vi "Initialize Global Stop.vi"(8 "error in":errorcluster, 11 "VS Plugin Inline Async API in":refnum<class "VS Plugin Inline Async API.lvclass">) -> (0 "error out":errorcluster, 3 "VS Plugin Inline Async API out":refnum<class "VS Plugin Inline Async API.lvclass">)   [LabVIEW 2024, in "VS Plugin Inline Async API.lvlib" / "VS Plugin Inline Async API.lvclass"]
uses:
  VS Plugin Inline Async API.lvclass
  VS Plugin Inline Async API.lvclass/VS Plugin Inline Async API.ctl
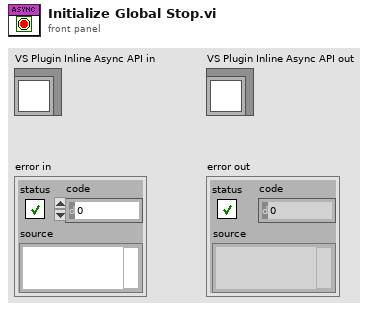
[diagram p1: front panel]
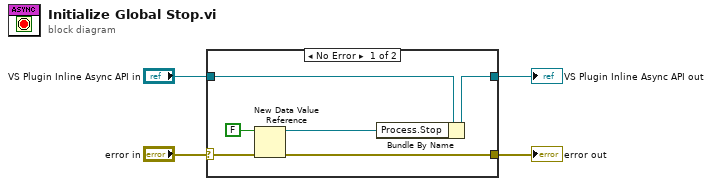
[diagram p0: block diagram]
diagram:
  n1 = case shown="No Error" "error in" {
    selector: "error in" -> [w10 w12]
    tunnel: [w9 w12] -> w3
    tunnel: "VS Plugin Inline Async API in" -> [w7 w11]
    tunnel: [w6 w11] -> w1
    frame No Error {
      n2 = New Data Value Reference(data value=FALSE, error in=w10) -> (data value reference=w5:refnum<data-value>, error out=w9:errorcluster)
      n3 = Bundle By Name(cluster=w7, "Process.Stop"=w5) -> (w6:refnum<class "VS Plugin Inline Async API.lvclass">)
    }
    frame Error {
    }
  }
  "error out" <- w3
  "VS Plugin Inline Async API out" <- w1
